vi "State_Machine.vi"(8 "error in (no error)":errorcluster caption="entrée d'erreur (pas d'erreur)", 11 "Get_Voltage en entrée":refnum<class "Zigbee_Remove_From_Network.lvclass">) -> (0 "error out":errorcluster caption="sortie d'erreur", 2 "Json_String":string, 3 "Get_Voltage en sortie":refnum<class "Zigbee_Remove_From_Network.lvclass">)   [LabVIEW 2020, in "Library Test.lvlib" / "Zigbee_Remove_From_Network.lvclass"]
uses:
  Zigbee_Remove_From_Network.lvclass
  C:/Users/ngarcin/OneDrive - Altyor/Standard TB/Suite TB45/Class/Test/Zigbee_Send_Command_UART/Zigbee_Send_Command_UART.lvclass
  C:/Users/ngarcin/OneDrive - Altyor/Standard TB/Suite TB45/Class/Test/Test (Default)/Test (Default).lvclass
  Commun VI/TypeDef/Variable Printable.ctl
  Zigbee_Send_Command_UART/Zigbee_Send_Command_UART.lvclass
  Commun VI/Library Commun.lvlib
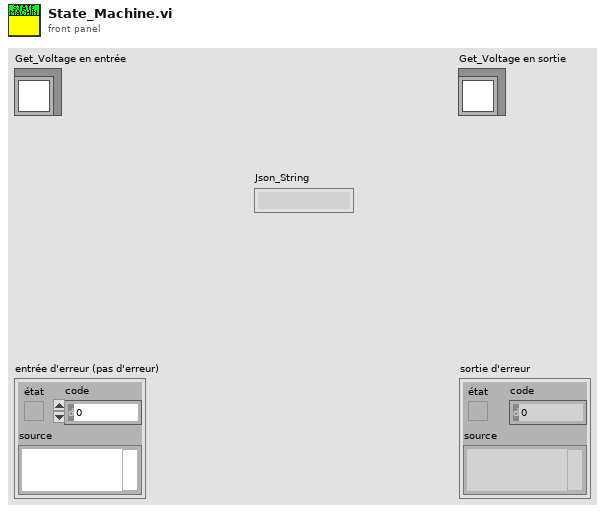
[diagram p1: front panel]
types:
  T1 = typedef "Variable Printable.ctl" = string
  T2 = enum16{"Get Variable", "Get All Variables", "Set Variable", "Delete Variable", "Delete All Variable"}
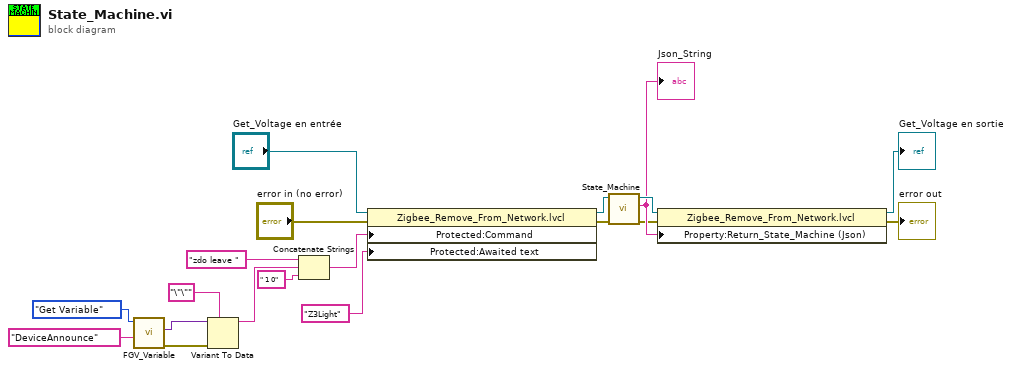
[diagram p0: block diagram]
diagram:
  n1 = call "FGV_Variable.vi"("Variable"=T1 "DeviceAnnounce", "Function"=T2."Get Variable") -> ("error out"=w4:errorcluster, "Data Out"=w3:variant)  [unwired: 7 in, 1 out]
  n2 = Variant To Data(error in=w4, type="\"\"", Variant=w3) -> (data=w1:string)  [unwired: 1 out]
  n3 = Concatenate Strings("zdo leave " ("Command"), w1, " 1 0" ("string")) -> (w7:string)
  n4 = property class="Zigbee_Remove_From_Network.lvcl"(reference="Get_Voltage en entrée", error in="error in (no error)", "Protected:Command"=w7, "Protected:Awaited text"="Z3Light" ("Awaited text")) -> (reference out=w19:refnum<class "Zigbee_Remove_From_Network.lvclass">, error out=w18:errorcluster)
  n5 = call-parent "State_Machine.vi"("error in (no error)"=w18, "Send_Frame en entrée"=w19) -> ("error out"=w11:errorcluster, "Json_String"=w13:string, "Send_Frame en sortie"=w14:refnum<class "Zigbee_Remove_From_Network.lvclass">)  [unwired: 7 in]
  "Json_String" <- w13
  n6 = property class="Zigbee_Remove_From_Network.lvcl"(reference=w14, error in=w11, "Property:Return_State_Machine (Json)"=w13) -> (reference out=→"Get_Voltage en sortie":refnum<class "Zigbee_Remove_From_Network.lvclass">, error out=→"error out":errorcluster)
